vi "DVRtoRef--SMO.vi"(10 "Ref":T1) -> (2 "Ref":u64 format="%016x")   [LabVIEW 2021, in "SMO.lvclass"]
uses:
  SMO.lvclass
  Typedefs/PrivateData--Ref.ctl
  Typedefs/PrivateData--Cluster.ctl
  Typedefs/Parent Call--Enum.ctl
  Typedefs/RegisteredProcessData--Cluster.ctl
  Typedefs/Process Error Notification--Cluster.ctl
  Typedefs/Protected Events.ctl
  Typedefs/StopProcessEventData--Cluster.ctl
  Typedefs/AbortProcessEventData--Cluster.ctl
  Typedefs/SMO Dependency Event--Cluster.ctl
  Typedefs/SMO Dependency Event--Enum.ctl
  Typedefs/Public Events.ctl
  Typedefs/SMOState --Enum.ctl
  Typedefs/Reserve State--Enum.ctl
  Typedefs/Accessibility--Cluster.ctl
  SMO.lvclass/SMO.ctl
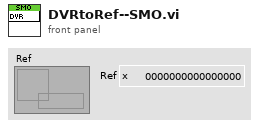
[diagram p1: front panel]
types:
  T1 = typedef "SMO.lvclass/PrivateData--Ref.ctl" = refnum<data-value>
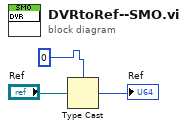
[diagram p0: block diagram]
diagram:
  n1 = Type Cast(type=u64 0 ("Ref"), x="Ref") -> (*(type *) &x=→"Ref":u64)
